vi "command array to mask (U8).vi"(11 "Array In":dbl[](array[numeric])) -> (3 "mask":u8)   [LabVIEW 2016, in "Scan Engine Custom Device.lvlib" / "DS402.lvlib"]
uses:
  DS402.lvlib
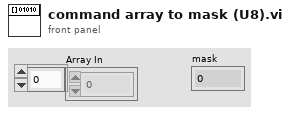
[diagram p1: front panel]
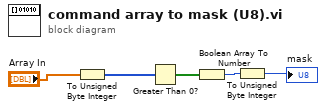
[diagram p0: block diagram]
diagram:
  n1 = To Unsigned Byte Integer(number="Array In") -> (unsigned 8bit integer=w5:u8[])
  n2 = Greater Than 0?(x=w5) -> (x > 0?=w4:bool[])
  n3 = Boolean Array To Number(Boolean array=w4) -> (number=w3:u32)
  n4 = To Unsigned Byte Integer(number=w3) -> (unsigned 8bit integer=→"mask":u8)
